vi "Test Write and Read.vi"(8 "error in (no error)":errorcluster) -> (0 "error out":errorcluster)   [LabVIEW 2009]
uses:
  Classes/Integer Dictionary.lvclass
  classes/Test/Test.lvclass
  classes/Assert/Assert.lvclass
panel:
  # "See block diagram"
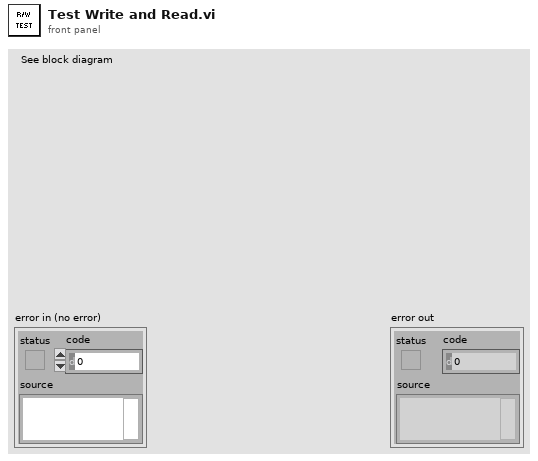
[diagram p1: front panel]
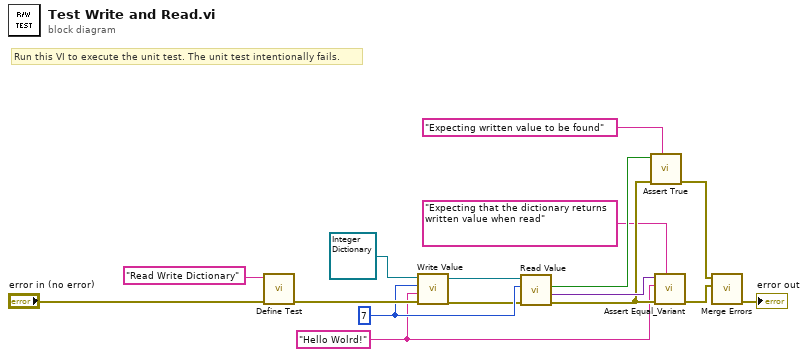
[diagram p0: block diagram]
diagram:
  w2 = "Hello Wolrd!"
  w11 = 7 ("Key")
  # "Run this VI to execute the unit test. The unit test intentionally fails."
  n1 = call "Define Test.vi"("error in (no error)"="error in (no error)", "Label (VI Title)"="Read Write Dictionary") -> ("error out"=w13:errorcluster)  [unwired: 9 in]
  n2 = call "Write Value.vi"("error in (no error)"=w13, "Value"=w2, "Key"=w11, "Integer Dictionary in"=refnum<class "Integer Dictionary.lvclass"> refnum) -> ("error out"=w10:errorcluster, "Integer Dictionary out"=w12:refnum<class "Integer Dictionary.lvclass">)  [unwired: 5 in, 1 out]
  n3 = call "Read Value.vi"("error in (no error)"=w10, "Key"=w11, "Integer Dictionary in"=w12) -> ("error out"=w7:errorcluster, "Value"=w9:variant, "found?"=w8:bool)  [unwired: 5 in, 1 out]
  n4 = call "Assert True.vi"("Label"="Expecting written value to be found", "error in (no error)"=w7, "True?"=w8) -> ("error out"=w4:errorcluster)  [unwired: 8 in]
  n5 = call "Assert Equal_Variant.vi"("Label"="Expecting that the dictionary returns written value when read", "error in (no error)"=w7, "Y"=w2, "X"=w9) -> ("error out"=w3:errorcluster)  [unwired: 7 in]
  n6 = call <vilib>:"Merge Errors.vi"("error in 2 (no error)"=w3, "error in 1 (no error)"=w4) -> ("error out"=→"error out":errorcluster)  [unwired: 5 in]
